vi "OL.vi"(11 "CMD_OL":T3) -> (3 "SM Status_OUT":T1)   [LabVIEW 2017, in "TemplateOverlord.lvlib"]
uses:
  TemplateOverlord.lvlib
  ENUM_State.ctl
  Cluster_CMD to OL Data.ctl
  ENUM_OL Cmd Select.ctl
  ENUM_Action.ctl
  Cluster_OL Status.ctl
  Globals/Global_STOP.vi
panel:
  out "Action":T2
  out "Current State":T5
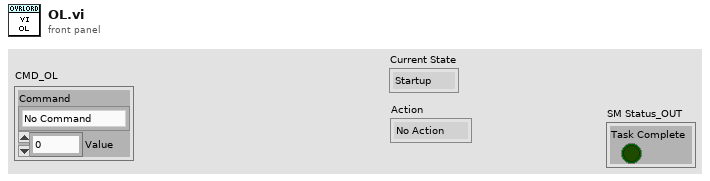
[diagram p1: front panel]
types:
  T1 = typedef "TemplateOverlord.lvlib/Cluster_OL Status.ctl" = cluster{"Task Complete":bool}
  T2 = typedef "TemplateOverlord.lvlib/ENUM_Action.ctl" = enum16{"No Action", "Reset Time", "Reset All", "Stop Action", "Set Action"}
  T3 = typedef "TemplateOverlord.lvlib/Cluster_CMD to OL Data.ctl" = cluster{"Command":T4, "Value":dbl}
  T4 = typedef "TemplateOverlord.lvlib/ENUM_OL Cmd Select.ctl" = enum16{"No Command", "Stop", "Go"}
  T5 = typedef "TemplateOverlord.lvlib/ENUM_State.ctl" = enum16{"Startup", "Idle", "Run", "Shutdown"}
  T6 = cluster{"Actions":T2[], "State":T5, "Current Time":timestamp, "Start Time":timestamp, "Loop Time (ms)":u32, "CMD_OL":T3, "OL Status_OUT":T1}
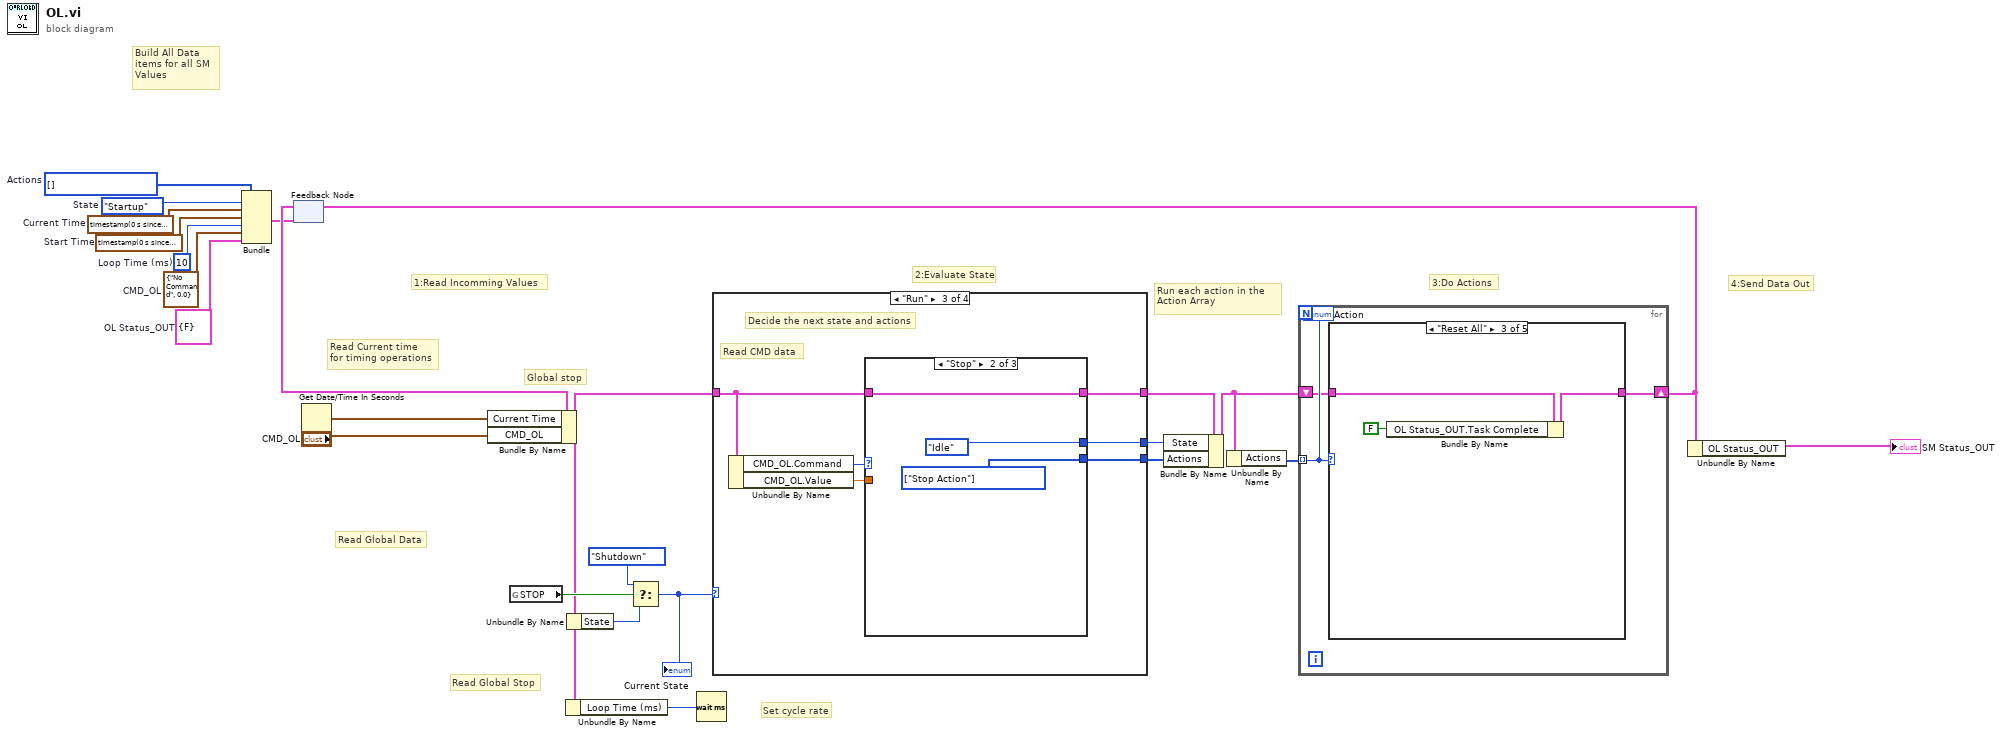
[diagram p0: block diagram]
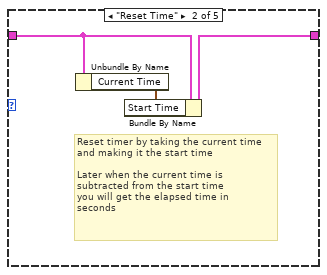
[diagram p3: hidden frame]
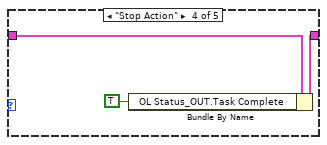
[diagram p4: hidden frame]
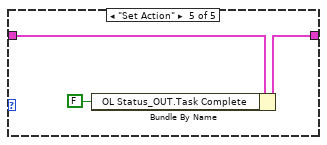
[diagram p5: hidden frame]
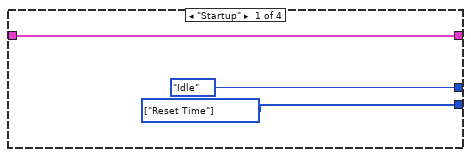
[diagram p6: hidden frame]
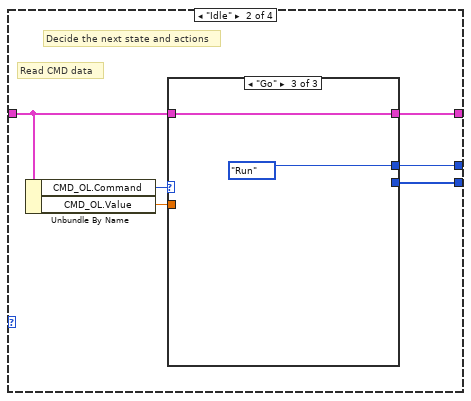
[diagram p7: hidden frame]
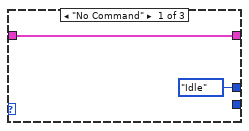
[diagram p8: hidden frame]
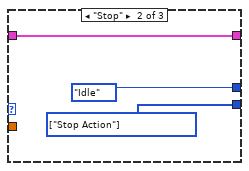
[diagram p9: hidden frame]
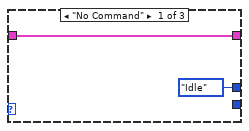
[diagram p10: hidden frame]
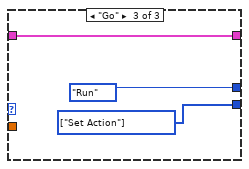
[diagram p11: hidden frame]
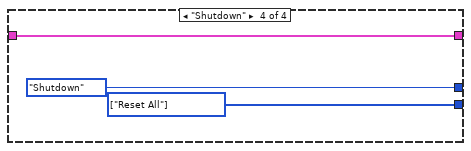
[diagram p12: hidden frame]
diagram:
  w18 = T1 {"Task Complete"=FALSE}  # OL Status_OUT
  w19 = T3 {"Command"=enum."No Command", "Value"=0.0}  # CMD_OL
  w20 = u32 10  # Loop Time (ms)
  w21 = T2[] [] items=["No Action", "Reset Time", "Reset All", "Stop Action", "Set Action"]  # Actions
  w22 = timestamp(0 s since 1904-01-01)  # Start Time
  w23 = timestamp(0 s since 1904-01-01)  # Current Time
  w24 = ENUM_State."Startup"  # State
  # "Read Global Data"
  # "Set cycle rate"
  # "Read Current time\nfor timing operations"
  # "Run each action in the Action Array"
  # "Read Global Stop"
  # "1:Read Incomming Values"
  # "2:Evaluate State"
  # "3:Do Actions"
  # "4:Send Data Out"
  # "Global stop"
  # "Build All Data items for all SM Values"
  n1 = Bundle("Actions"=w21, "State"=w24, "Current Time"=w23, "Start Time"=w22, "Loop Time (ms)"=w20, "CMD_OL"=w19, "OL Status_OUT"=w18) -> (w15:T6)  [unwired: 1 in]
  n2 = feedback #1(w15) -> (w16:T6)
  n3 = Get Date/Time In Seconds() -> (seconds since 1Jan1904=w13:timestamp)
  n4 = Bundle By Name(cluster=w16, "Current Time"=w13, "CMD_OL"="CMD_OL") -> (w3:T6)
  n5 = global read "Global_STOP.vi" "STOP"() -> (w8:bool)
  n6 = Unbundle By Name(w3) -> ("Loop Time (ms)"=w4:u32)
  n7 = Unbundle By Name(w3) -> ("State"=w6:T5)
  n8 = Select(t=ENUM_State."Shutdown" ("State"), s=w8, f=w6) -> (s? t:f=w5:T5)
  "Current State" <- w5
  n9 = Wait (ms)(milliseconds to wait=w4) -> ()  [unwired: 1 out]
  n10 = case shown="\"Run\"" w5 {
    tunnel: w3 -> [w27 w32 w45 w57]
    tunnel: [w27 w31 w44 w57] -> w11
    tunnel: [ENUM_State."Idle" ("State") w29 w42 ENUM_State."Shutdown" ("State")] -> w10
    tunnel: [w26 w28 w41 w55] -> w9
    frame "Startup" {
      w26 = T2[] [enum."Reset Time"] items=["No Action", "Reset Time", "Reset All", "Stop Action", "Set Action"] ("Actions")
    }
    frame "Idle" {
      # "Read CMD data"
      # "Decide the next state and actions"
      n11 = Unbundle By Name(w32) -> ("CMD_OL.Command"=w33:T4, "CMD_OL.Value"=w30:dbl)
      n12 = case shown="\"Go\"" w33 {
        tunnel: w32 -> [w35 w38 w40]
        tunnel: [w35 w38 w40] -> w31
        tunnel: w30 -> [_ _ _]
        tunnel: [ENUM_State."Idle" ("State") ENUM_State."Idle" ("State") ENUM_State."Run" ("State")] -> w29
        tunnel: [_ w36 _] -> w28
        frame "No Command" {
        }
        frame "Stop" {
          w36 = T2[] [enum."Stop Action"] items=["No Action", "Reset Time", "Reset All", "Stop Action", "Set Action"] ("Actions")
        }
        frame "Go" {
        }
      }
    }
    frame "Run" {
      # "Read CMD data"
      # "Decide the next state and actions"
      n13 = Unbundle By Name(w45) -> ("CMD_OL.Command"=w46:T4, "CMD_OL.Value"=w43:dbl)
      n14 = case shown="\"Stop\"" w46 {
        tunnel: w45 -> [w48 w51 w54]
        tunnel: [w48 w51 w54] -> w44
        tunnel: w43 -> [_ _ _]
        tunnel: [ENUM_State."Idle" ("State") ENUM_State."Idle" ("State") ENUM_State."Run" ("State")] -> w42
        tunnel: [_ w49 w52] -> w41
        frame "No Command" {
        }
        frame "Stop" {
          w49 = T2[] [enum."Stop Action"] items=["No Action", "Reset Time", "Reset All", "Stop Action", "Set Action"] ("Actions")
        }
        frame "Go" {
          w52 = T2[] [enum."Set Action"] items=["No Action", "Reset Time", "Reset All", "Stop Action", "Set Action"] ("Actions")
        }
      }
    }
    frame "Shutdown" {
      w55 = T2[] [enum."Reset All"] items=["No Action", "Reset Time", "Reset All", "Stop Action", "Set Action"] ("Actions")
    }
  }
  n15 = Bundle By Name(cluster=w11, "State"=w10, "Actions"=w9) -> (w12:T6)
  n16 = Unbundle By Name(w12) -> ("Actions"=w14:T2[])
  n17 = for {
    tunnel: w14 -> [w60] mode=indexing
    shift-right: [w59] -> w17
    shift-left: w12 -> [w58]
    n18 = case shown="\"Reset All\"" w60 {
      tunnel: w58 -> [w61 w64 w67 w70 w73]
      tunnel: [w61 w63 w66 w69 w72] -> w59
      frame "No Action" {
      }
      frame "Reset Time" {
        # "Reset timer by taking the current time\nand making it the start time\n\nLater when the current time is \nsubtracted from the start time\nyou will get the elapsed time in \nseconds"
        n19 = Unbundle By Name(w64) -> ("Current Time"=w62:timestamp)
        n20 = Bundle By Name(cluster=w64, "Start Time"=w62) -> (w63:T6)
      }
      frame "Reset All" {
        n21 = Bundle By Name(cluster=w67, "OL Status_OUT.Task Complete"=FALSE) -> (w66:T6)
      }
      frame "Stop Action" {
        n22 = Bundle By Name(cluster=w70, "OL Status_OUT.Task Complete"=TRUE) -> (w69:T6)
      }
      frame "Set Action" {
        n23 = Bundle By Name(cluster=w73, "OL Status_OUT.Task Complete"=FALSE) -> (w72:T6)
      }
    }
    "Action" <- w60
  }
  n24 = feedback-in #1(w17) -> ()
  n25 = Unbundle By Name(w17) -> ("OL Status_OUT"=→"SM Status_OUT":T1)
